vi "setUp.vi"(8 "error in (no error)":errorcluster) -> (0 "error out":errorcluster, 2 "connection ID":refnum<k5>, 3 "session":T1, 5 "fixture":refnum<class "Server Fixture.lvclass">)   [LabVIEW 2013, in "libssh2_integration_tests.lvlib"]
uses:
  libssh2_integration_tests.lvlib
  libssh2/Session Refnum.ctl
  Server Fixture/Server Fixture.lvclass
  Server Fixture/Server Fixture.lvclass/Server Fixture.ctl
  Server Fixture/Read User Private Key File.vi
  Server Fixture/Read User Public Key File.vi
  Server Fixture/Read User Name.vi
  Server Fixture/Read User Private Key Passphrase.vi
  Server Fixture/Read Server Address.vi
  Server Fixture/Read Server Port.vi
  libssh2/libssh2_init_default.vi
  libssh2/libssh2_session_handshake_tcp.vi
  libssh2/libssh2.lvlib
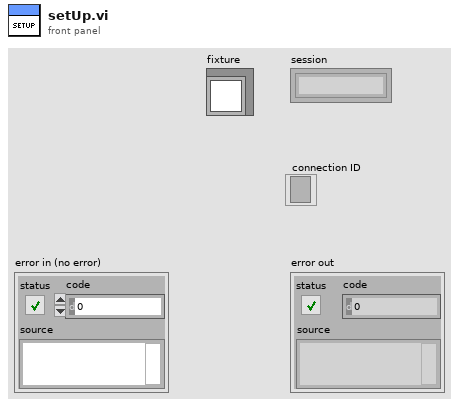
[diagram p1: front panel]
types:
  T1 = typedef "libssh2.lvlib/Session Refnum.ctl" = refnum<k1>
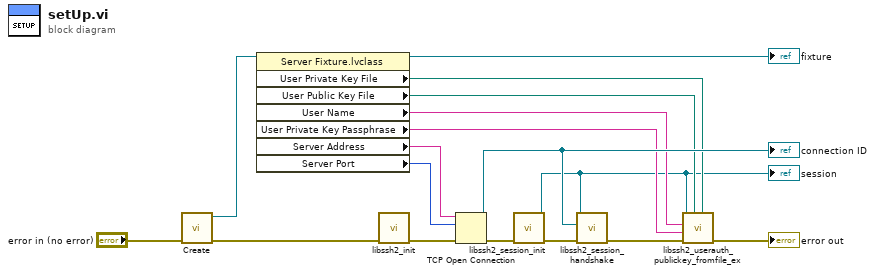
[diagram p0: block diagram]
diagram:
  n1 = call "Create.vi"("error in (no error)"="error in (no error)") -> ("error out"=w7:errorcluster, "Server Fixture"=w6:refnum<class "Server Fixture.lvclass">)  [unwired: 9 in]
  n2 = property on="Property Node" class="Server Fixture.lvclass"(reference=w6) -> (reference out=→"fixture":refnum<class "Server Fixture.lvclass">, "User Private Key File"=w13:path, "User Public Key File"=w14:path, "User Name"=w12:string, "User Private Key Passphrase"=w11:string, "Server Address"=w5:string, "Server Port"=w4:u16)  [unwired: 1 in, 1 out]
  n3 = call-poly "libssh2_init.vi"("error in (no error)"=w7) -> ("error out"=w16:errorcluster)  [unwired: 10 in]
  n4 = TCP Open Connection(address=w5, remote port or service name=w4, error in (no error)=w16) -> (connection ID=w15:refnum<k5>, error out=w17:errorcluster)  [unwired: 2 in]
  "connection ID" <- w15
  n5 = call "libssh2_session_init.vi"("error in (no error)"=w17) -> ("error out"=w8:errorcluster, "session"=w9:T1)  [unwired: 9 in]
  "session" <- w9
  n6 = call-poly "libssh2_session_handshake.vi"("error in (no error)"=w8, "tcp connection"=w15, "session"=w9) -> ("error out"=w10:errorcluster)  [unwired: 8 in]
  n7 = call "libssh2_userauth_publickey_fromfile_ex.vi"("private key"=w13, "public key"=w14, "error in (no error)"=w10, "passphrase"=w11, "username"=w12, "session"=w9) -> ("error out"=→"error out":errorcluster)  [unwired: 5 in]
